vi "command engine read async FIFOs.vi"(8 "error in (no error)":errorcluster, 9 "State Variables":T5, 10 "Parameters":T8 {"Compiled"."External Channels"."Channels" format="%.0x"; "Compiled"."External Channels"."Triggers" format="%.0x"}, 11 "Global Variables":T1) -> (0 "error out":errorcluster, 1 "State Variables out":T5, 2 "Parameters out":T8 {"Compiled"."External Channels"."Channels" format="%.0x"; "Compiled"."External Channels"."Triggers" format="%.0x"}, 3 "Global Variables out":T1)   [LabVIEW 2019, in "Instrument Addon Engine.lvlib"]
uses:
  Instrument Addon Engine.lvlib
  Types/Commands RT Configuration Cluster.ctl
  Protocols.lvlibp/Protocol Parent/Protocol Parent.lvclass
  Shared/Types/Compiled Settings.ctl
  Shared/Types/Command Parameters.ctl
  Shared/Types/Linked Channel Cluster.ctl
  Shared/Types/Command Channel Indeces.ctl
  Shared/Types/Command Channel Index.ctl
  Shared/Types/Response RT Configuration Cluster.ctl
  Shared/Types/Response Parameters.ctl
  Shared/Types/Response Wait Type.ctl
  Shared/Types/Message Parameters.ctl
  Shared/Types/Message Generation Type.ctl
  Shared/Types/External Trigger Refs.ctl
  <vilib>/NI VeriStand/Custom Device API/Data Reference.ctl
  Protections.lvlibp/Parent Protection/Protection.lvclass
  Types/Engine State Variables.ctl
  <vilib>/NI/NIVS Inline Async API/_VS Inline Async API/Process/Process.lvclass
  <vilib>/NI/NIVS Addon Network Comm/Engine/VeriStand Comm.lvclass
  <vilib>/NI/NIVS Inline Async API/_Data Access Engine/Data Access Engine/Types/Write.DVR.ctl
  <vilib>/NI/NIVS Inline Async API/_Data Access Engine/Access Type Classes/Write/Write.lvclass
  <vilib>/NI/NIVS Inline Async API/_Data Access Engine/Data Access Engine/Types/Read.DVR.ctl
  <vilib>/NI/NIVS Inline Async API/_Data Access Engine/Access Type Classes/Read/Read.lvclass
  <vilib>/NI/NIVS Inline Async API/_Data Access Engine/Data Access Engine/Types/ReadWrite.DVR.ctl
  <vilib>/NI/NIVS Inline Async API/_Data Access Engine/Access Type Classes/ReadWrite/ReadWrite.lvclass
  Types/command engine global variables.ctl
  <vilib>/NI/AMC/Message Queue.ctl
  <vilib>/NI/AMC/Message.ctl
  <vilib>/NI/Tools/Keyed Array/KeyedArray.ctl
  <vilib>/NI/NIVS Inline Async API/_Data Access Engine/Access Type Classes/ReadWrite/ReadWrite.lvclass/ReadWrite.ctl
  <vilib>/NI/NIVS Inline Async API/_Data Access Engine/Access Type Classes/Read/Read.lvclass/Read.ctl
  <vilib>/NI/NIVS Inline Async API/_Data Access Engine/Data Access Engine/Methods/ReadWrite.Data.Read.vi
  <vilib>/NI/NIVS Inline Async API/_Data Access Engine/Data Access Engine/Methods/Read.Data.vi
  <vilib>/NI/NIVS Inline Async API/_Data Access Engine/Data Access Engine/Methods/Read.Data.Detect.vi
  <vilib>/NI/NIVS Inline Async API/_Data Access Engine/Access Type Classes/ReadWrite/ReadWrite.ProcessData.Read.vi
  <vilib>/NI/NIVS Inline Async API/_Data Access Engine/Access Type Classes/Read/Read.ProcessData.vi
  <vilib>/NI/NIVS Inline Async API/_Data Access Engine/Access Type Classes/Read/Read.ProcessData.Detect.vi
  <vilib>/NI/NIVS Inline Async API/_Data Access Engine/Data Access Engine/Data Access Engine.lvclass
  Shared/Instrument Addon Shared.lvlib
  <vilib>/NI VeriStand/Custom Device API/Custom Device API.lvlib
  <vilib>/NI/Tools/Keyed Array/Tools_KeyedArray.lvlib
  <vilib>/NI/AMC/AMC.lvlib
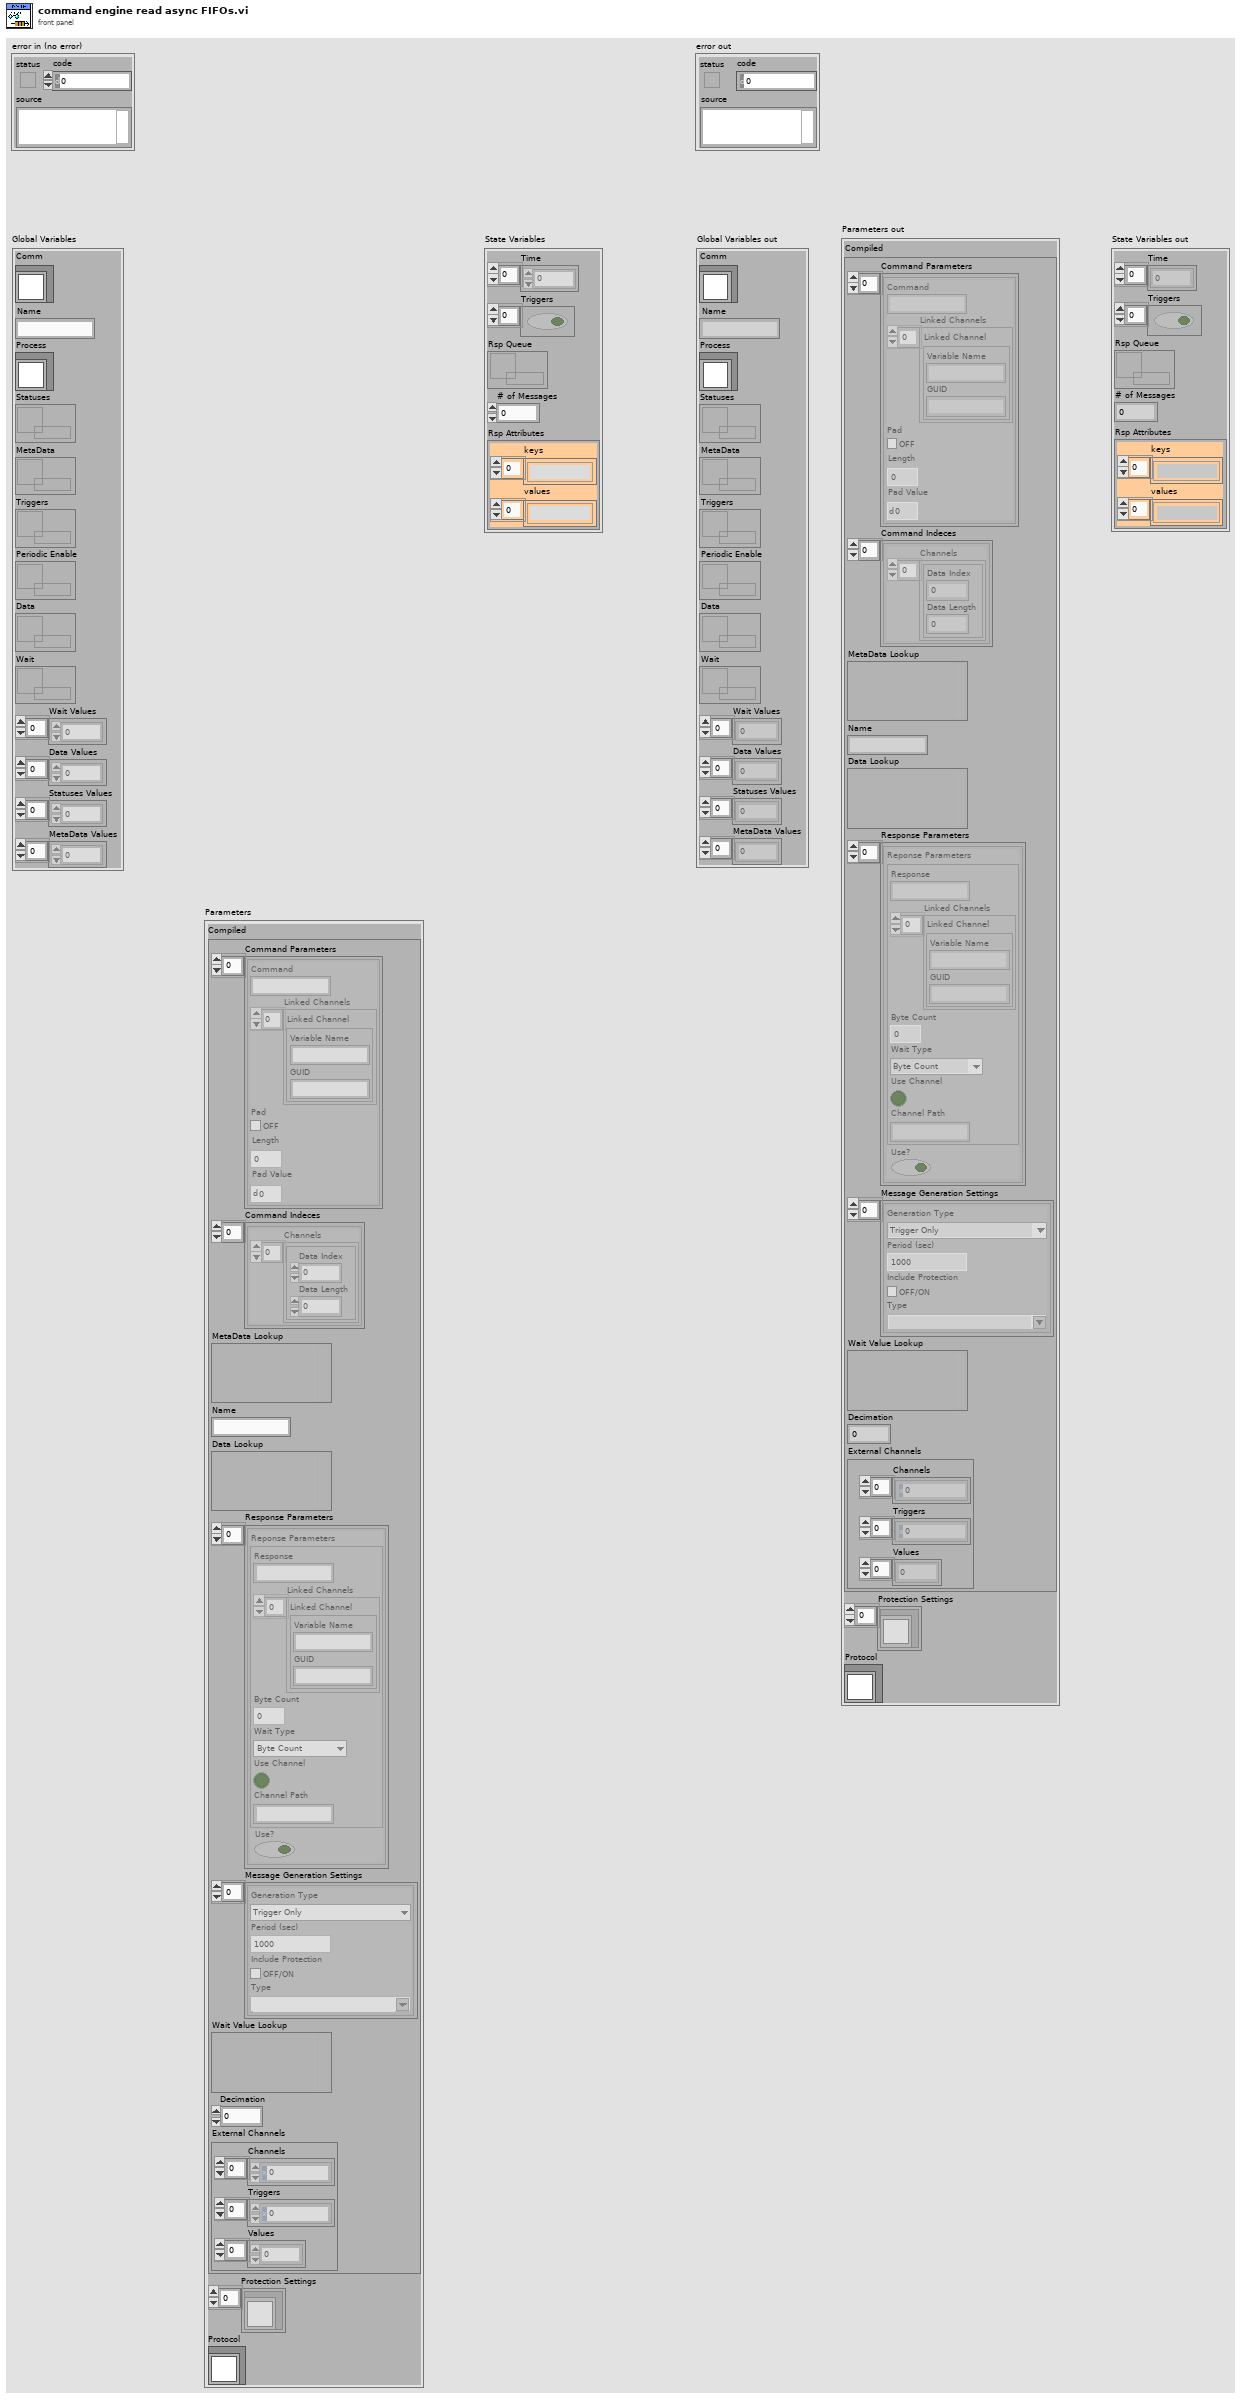
[diagram p1: front panel]
types:
  T1 = typedef "Instrument Addon Engine.lvlib/Engine State Variables.ctl" = cluster{"Comm":refnum<class "VeriStand Comm.lvclass">, "Name":string, "Process":refnum<class "Process.lvclass">, "Statuses":T2, "MetaData":T3, "Triggers":T4, "Periodic Enable":T3, "Data":T2, "Wait":T3, "Wait Values":dbl[], "Data Values":dbl[], "Statuses Values":dbl[], "MetaData Values":dbl[]}
  T2 = typedef "Data Access Engine.lvlib/Data Access Engine.lvclass/Write.DVR.ctl" = refnum<data-value>
  T3 = typedef "Data Access Engine.lvlib/Data Access Engine.lvclass/Read.DVR.ctl" = refnum<data-value>
  T4 = typedef "Data Access Engine.lvlib/Data Access Engine.lvclass/ReadWrite.DVR.ctl" = refnum<data-value>
  T5 = typedef "Instrument Addon Engine.lvlib/command engine global variables.ctl" = cluster{"Time":u32[], "Triggers":bool[], "Rsp Queue":T6, "# of Messages":i32, "Rsp Attributes":T7}
  T6 = typedef "AMC.lvlib/Message Queue.ctl" = refnum<queue>
  T7 = typedef "Tools_KeyedArray.lvlib/KeyedArray.ctl" = cluster{"keys":string[], "values":string[]}
  T8 = typedef "Instrument Addon Engine.lvlib/Commands RT Configuration Cluster.ctl" = cluster{"Compiled":T9, "Protection Settings":refnum<class "Protection.lvclass">[], "Protocol":refnum<class "Protocol Parent.lvclass">}
  T9 = typedef "Instrument Addon Shared.lvlib/Compiled Settings.ctl" = cluster{"Command Parameters":T10[], "Command Indeces":T12[], "MetaData Lookup":variant, "Name":string, "Data Lookup":variant, "Response Parameters":T14[], "Message Generation Settings":T17[], "Wait Value Lookup":variant, "Decimation":u32, "External Channels":T19}
  T10 = typedef "Instrument Addon Shared.lvlib/Command Parameters.ctl" = cluster{"Command":string, "Linked Channels":T11[], "Pad":bool, "Length":u32, "Pad Value":u8}
  T11 = typedef "Instrument Addon Shared.lvlib/Linked Channel Cluster.ctl" = cluster{"Variable Name":string, "GUID":string}
  T12 = typedef "Instrument Addon Shared.lvlib/Command Channel Indeces.ctl" = cluster{"Channels":T13[]}
  T13 = typedef "Instrument Addon Shared.lvlib/Command Channel Index.ctl" = cluster{"Data Index":i32, "Data Length":i32}
  T14 = typedef "Instrument Addon Shared.lvlib/Response RT Configuration Cluster.ctl" = cluster{"Reponse Parameters":T15, "Use?":bool}
  T15 = typedef "Instrument Addon Shared.lvlib/Response Parameters.ctl" = cluster{"Response":string, "Linked Channels":T11[], "Type Value":dbl, "Wait Type":T16, "Use Channel":bool, "Channel Path":string}
  T16 = typedef "Instrument Addon Shared.lvlib/Response Wait Type.ctl" = enum16{"Byte Count", "Wait sec"}
  T17 = typedef "Instrument Addon Shared.lvlib/Message Parameters.ctl" = cluster{"Generation Type":T18, "Period":dbl, "Include Protection":bool, "Type":string}
  T18 = typedef "Instrument Addon Shared.lvlib/Message Generation Type.ctl" = enum16{"Trigger Only", "Periodic & Trigger", "Value Change & Trigger"}
  T19 = typedef "Instrument Addon Shared.lvlib/External Trigger Refs.ctl" = cluster{"Channels":T20[], "Triggers":T20[], "Values":dbl[]}
  T20 = typedef "Custom Device API.lvlib/Data Reference.ctl" = i32
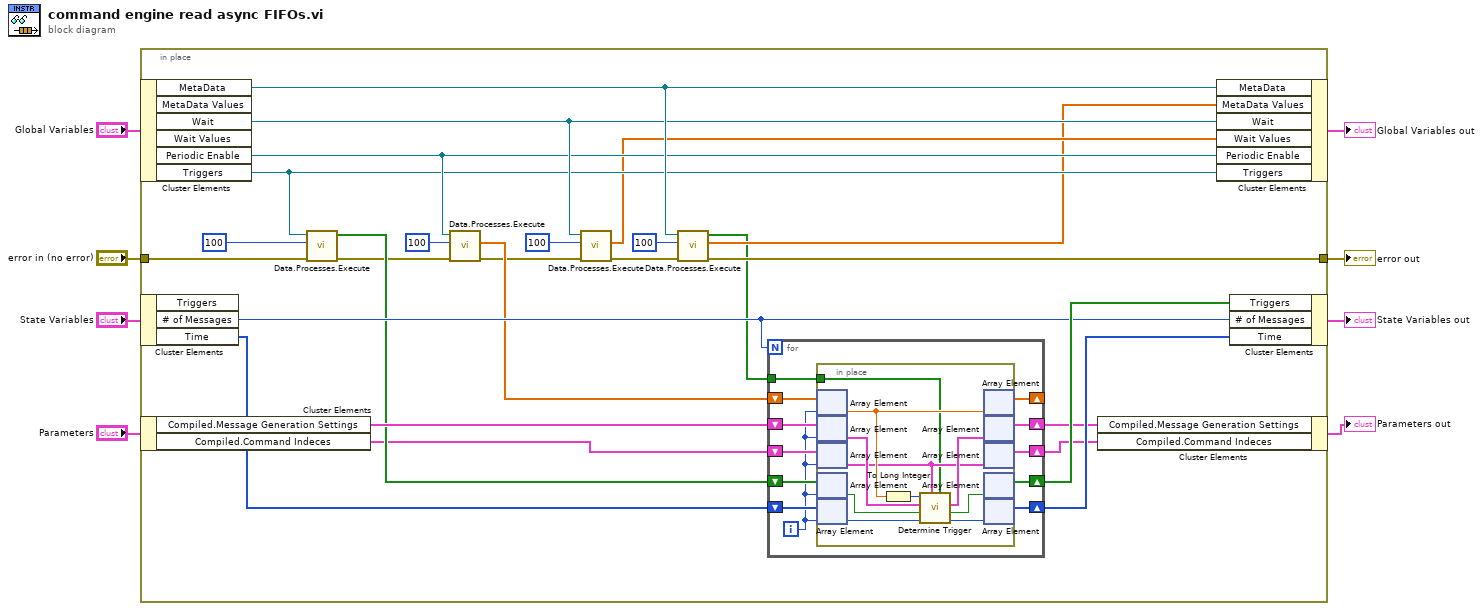
[diagram p0: block diagram]
diagram:
  n1 = in-place {
    in-place-border: [w18] -> w8
    in-place-border: "error in (no error)" -> [w27]
    n2 = in-place-cluster #1("Global Variables") -> ("MetaData"=w17:T3, "Wait"=w16:T3, "Periodic Enable"=w15:T3, "Triggers"=w14:T4)  [unwired: 2 out]
    n3 = in-place-cluster #2("State Variables") -> ("# of Messages"=w29:i32, "Time"=w33:u32[])  [unwired: 1 out]
    n4 = in-place-cluster #3("Parameters") -> ("Compiled.Message Generation Settings"=w34:T17[], "Compiled.Command Indeces"=w11:T12[])
    n5 = call-poly <vilib>:"Data.Processes.Execute.vi"("error in (no error)"=w27, "timeout ms"=100 ("timeout in ms (0)"), "Ref"=w14) -> ("error out"=w24:errorcluster, "Detect?"=w28:bool[])  [unwired: 5 in, 2 out]
    n6 = call-poly <vilib>:"Data.Processes.Execute.vi"("error in (no error)"=w24, "timeout ms"=100 ("timeout in ms (0)"), "Ref"=w15) -> ("error out"=w21:errorcluster, "Values"=w23:dbl[])  [unwired: 6 in, 1 out]
    n7 = call-poly <vilib>:"Data.Processes.Execute.vi"("error in (no error)"=w21, "timeout ms"=100 ("timeout in ms (0)"), "Ref"=w16) -> ("error out"=w20:errorcluster, "Values"=w13:dbl[])  [unwired: 6 in, 1 out]
    n8 = call-poly <vilib>:"Data.Processes.Execute.vi"("error in (no error)"=w20, "timeout ms"=100 ("timeout in ms (0)"), "Ref"=w17) -> ("error out"=w18:errorcluster, "Values"=w12:dbl[], "Detect?"=w9:bool[])  [unwired: 5 in, 1 out]
    n9 = for {
      N: w29 -> [_]
      shift-right: [w45] -> w30
      shift-left: w34 -> [w46]
      shift-right: [w43] -> w31
      shift-left: w28 -> [w44]
      shift-right: [w39] -> w32
      shift-left: w33 -> [w42]
      shift-right: [w40] -> _
      shift-left: w23 -> [w41]
      shift-right: [w37] -> w10
      shift-left: w11 -> [w38]
      tunnel: w9 -> [w35]
      i -> [w36]
      n10 = in-place {
        in-place-border: w35 -> [w47]
        n11 = in-place-array #4(w41, w36) -> (w52:dbl)
        n12 = in-place-array #5(w46, w36) -> (w50:T17)
        n13 = in-place-array #6(w38, w36) -> (w48:T12)
        n14 = in-place-array #7(w44, w36) -> (w51:bool)
        n15 = in-place-array #8(w42, w36) -> (w55:u32)
        n16 = To Long Integer(number=w52) -> (32bit integer=w53:i32)
        n17 = call "Determine Trigger.vi"("Detect?"=w47, "Command Indeces"=w48, "Time Since Last Generation"=w55, "Trigger"=w51, "Message Parameters"=w50, "Enabled"=w53) -> ("Time Since Last Generation"=w54:u32, "Trigger"=w49:bool)  [unwired: 4 in]
        n18 = in-place-array #4(w52) -> (w40:dbl[])  [unwired: 1 out]
        n19 = in-place-array #5(w50) -> (w45:T17[])  [unwired: 1 out]
        n20 = in-place-array #6(w48) -> (w37:T12[])  [unwired: 1 out]
        n21 = in-place-array #7(w49) -> (w43:bool[])  [unwired: 1 out]
        n22 = in-place-array #8(w54) -> (w39:u32[])  [unwired: 1 out]
      }
    }
    n23 = in-place-cluster #3("Compiled.Message Generation Settings"=w30, "Compiled.Command Indeces"=w10) -> (→"Parameters out":T8)
    n24 = in-place-cluster #1("MetaData"=w17, "MetaData Values"=w12, "Wait"=w16, "Wait Values"=w13, "Periodic Enable"=w15, "Triggers"=w14) -> (→"Global Variables out":T1)
    n25 = in-place-cluster #2("Triggers"=w31, "# of Messages"=w29, "Time"=w32) -> (→"State Variables out":T5)
  }
  "error out" <- w8
